vi "Write Port.vi"(8 "error in (no error)":errorcluster, 10 "Port":u16, 11 "TcpSocket in":refnum<class "TcpSocket.lvclass">) -> (0 "error out":errorcluster, 3 "TcpSocket out":refnum<class "TcpSocket.lvclass">)   [LabVIEW 2022 SP3, in "TcpSocket.lvlib" / "TcpSocket.lvclass"]
uses:
  TcpSocket.lvclass
  TcpSocket.lvclass/TcpSocket.ctl
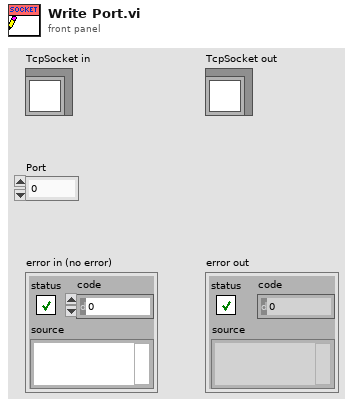
[diagram p1: front panel]
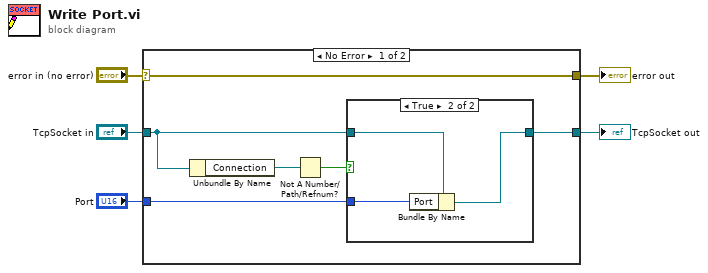
[diagram p0: block diagram]
diagram:
  n1 = case shown="No Error" "error in (no error)" {
    selector: "error in (no error)" -> [w11 w16]
    tunnel: [w11 w16] -> w4
    tunnel: [w10 w17] -> w3
    tunnel: "TcpSocket in" -> [w8 w17]
    tunnel: "Port" -> [w9 _]
    frame No Error {
      n2 = Unbundle By Name(w8) -> ("Connection"=w7:refnum<k5>)
      n3 = Not A Number/Path/Refnum?(number/path/refnum=w7) -> (NaN/Path/Refnum?=w6:bool)
      n4 = case shown="True" w6 {
        tunnel: [w12 w15] -> w10
        tunnel: w9 -> [_ w14]
        tunnel: w8 -> [w12 w13]
        frame False {
        }
        frame True {
          n5 = Bundle By Name(cluster=w13, "Port"=w14) -> (w15:refnum<class "TcpSocket.lvclass">)
        }
      }
    }
    frame Error {
    }
  }
  "error out" <- w4
  "TcpSocket out" <- w3
